vi "write command.vi"(8 "error in (no error)":errorcluster, 10 "command interface":T1={"command"=enum."Idle", "start time (ms)"=0, "Channel Indices"=[], "Scans per Sample"=1} {"Scans per Sample" min=1}, 11 "refnum in":refnum<k5>) -> (0 "error out":errorcluster, 3 "refnum out":refnum<k5>)   [LabVIEW 2012]
uses:
  DataServer/command cluster.ctl
  DataServer/command.ctl
panel:
  out "bytes written":i32
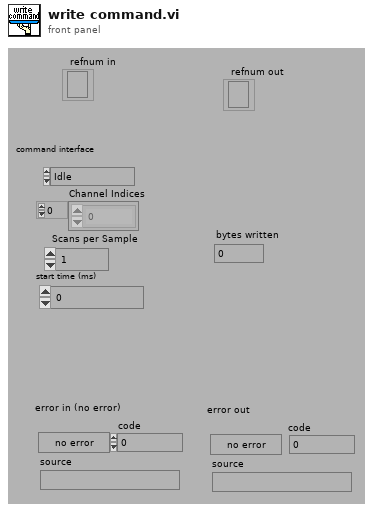
[diagram p1: front panel]
types:
  T1 = typedef "command cluster.ctl" = cluster{"command":T2, "start time (ms)":u32, "Channel Indices":i32[], "Scans per Sample":i32}
  T2 = typedef "command.ctl" = enum16{"Idle", "Send Data", "Send 1 Scan", "Logoff"}
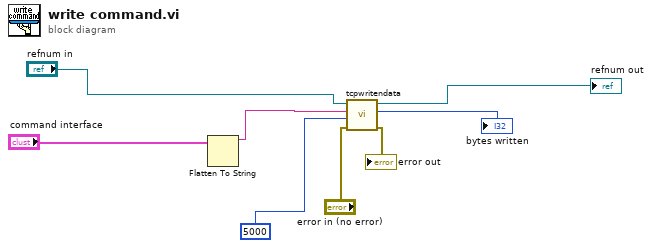
[diagram p0: block diagram]
diagram:
  n1 = Flatten To String(anything="command interface") -> (data string=w2:string)  [unwired: 3 in, 2 out]
  n2 = call "tcpwritendata.vi"("error in (no error)"="error in (no error)", "timeout ms (25000)"=5000, "data in"=w2, "refnum in"="refnum in") -> ("error out"=→"error out":errorcluster, "bytes written"=→"bytes written":i32, "refnum out"=→"refnum out":refnum<k5>)  [unwired: 5 in]
